vi "mlog2.vi"(4 "reference":refnum<vi>, 5 "String":string, 7 "error in":errorcluster) -> ()   [LabVIEW 2010]
uses:
  <vilib>/Utility/error.llb/DialogType.ctl
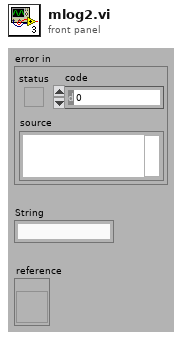
[diagram p1: front panel]
types:
  T1 = typedef "DialogType.ctl" = u16
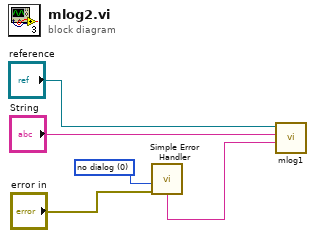
[diagram p0: block diagram]
diagram:
  w5 = T1 0 items=["no dialog", "OK message", "continue or stop message", "OK message + warnings", "continue/stop + warnings"] ("type of dialog (OK msg:1)")
  n1 = call <vilib>:"Simple Error Handler.vi"("type of dialog (OK msg:1)"=w5, "error in (no error)"="error in") -> ("message"=w1:string)  [unwired: 3 in, 4 out]
  n2 = call "mlog1.vi"("string2"=w1, "string1"="String", "message"="reference") -> ()  [unwired: 5 in]
